vi "mxwScript_Cmnd2Str_createControlsIndicators.vi"(8 "error in (no error)":errorcluster, 11 "data":variant) -> (0 "error out":errorcluster, 3 "outputString":string)   [LabVIEW 2020]
uses:
  codeGenAPISupport.llb/cgAPI_mxwScript_DrpTmplt_CreateControlsIndicatorsData.ctl
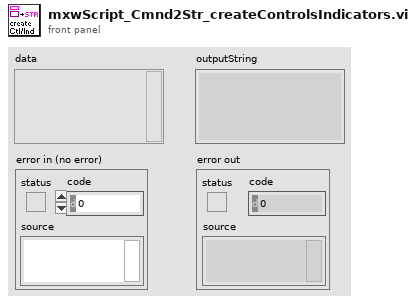
[diagram p1: front panel]
types:
  T1 = typedef "cgAPI_mxwScript_DrpTmplt_CreateControlsIndicatorsData.ctl" = cluster{"nodeLabel":string, "nodePattern":string, "diagramRef":refnum<vi>, "uniquify":bool, "createControls":bool, "createIndicators":bool, "templateIndex":i32}
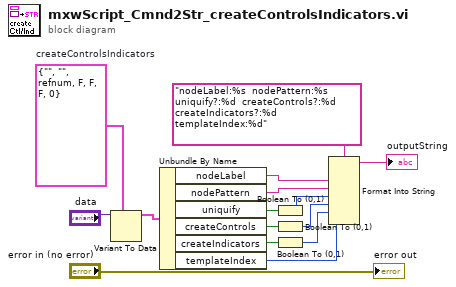
[diagram p0: block diagram]
diagram:
  w6 = T1 {"nodeLabel"="", "nodePattern"="", "diagramRef"=refnum, "uniquify"=FALSE, "createControls"=FALSE, "createIndicators"=FALSE, "templateIndex"=0}  # createControlsIndicators
  n1 = Variant To Data(type=w6, Variant="data") -> (data=w14:T1)  [unwired: 1 in, 1 out]
  n2 = Unbundle By Name(w14) -> ("nodeLabel"=w11:string, "nodePattern"=w9:string, "uniquify"=w8:bool, "createControls"=w10:bool, "createIndicators"=w3:bool, "templateIndex"=w1:i32)
  n3 = Boolean To (0,1)(Boolean=w8) -> (0, 1=w5:i16)
  n4 = Boolean To (0,1)(Boolean=w10) -> (0, 1=w4:i16)
  n5 = Boolean To (0,1)(Boolean=w3) -> (0, 1=w2:i16)
  n6 = Format Into String(format string="nodeLabel:%s  nodePattern:%s  uniquify?:%d  createControls?:%d  createIndicators?:%d  templateIndex:%d", w11, w9, w5, w4, w2, w1) -> (resulting string=→"outputString":string)  [unwired: 2 in, 1 out]
  "error out" <- "error in (no error)"
